vi "3D_to_2D_Sum_sub.vi"(1 "3D array":ext[][][](array[numeric])=array5x10x784[39200 elements]) -> (0 "2D_sum array":ext[][](array[numeric]))   [LabVIEW 2021]
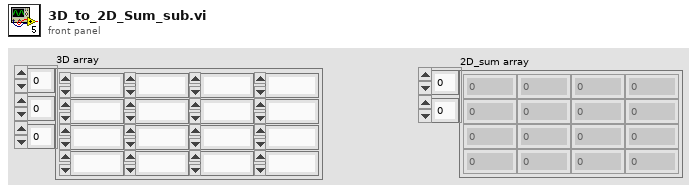
[diagram p1: front panel]
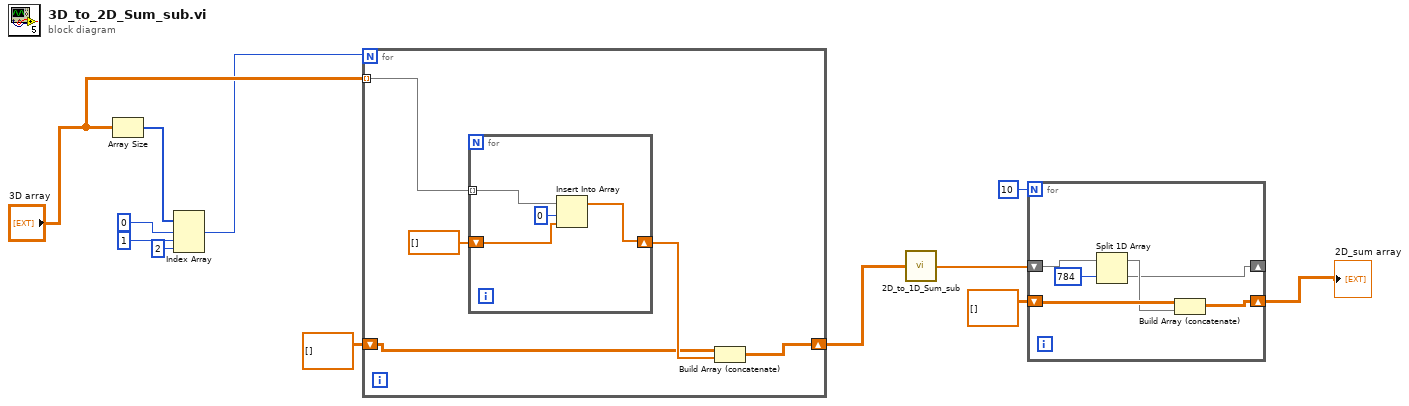
[diagram p0: block diagram]
diagram:
  n1 = Array Size(array="3D array") -> (size(s)=w12:i32[])
  n2 = Index Array(array=w12, index #1=0 ("인덱스"), index #2=1 ("인덱스"), index #3=2 ("인덱스")) -> (element #1=w7:i32)  [unwired: 2 out]
  n3 = for {
    N: w7 -> [_]
    tunnel: "3D array" -> [w16] mode=indexing
    shift-right: [w13] -> w5
    shift-left: ext[][] [] -> [w14]
    n4 = for {
      tunnel: w16 -> [w21] mode=indexing
      shift-right: [w20] -> w15
      shift-left: ext[] [] ("배열 2") -> [w19]
      n5 = Insert Into Array(array=w21, index=0 ("인덱스"), new element=w19) -> (w20:ext[])
    }
    n6 = Build Array (concatenate)(w14, w15) -> (w13:ext[][])
  }
  n7 = call "2D_to_1D_Sum_sub.vi"("2D array"=w5) -> ("1D array"=w2:ext[])
  n8 = for {
    N: 10 -> [_]
    shift-right: [w26] -> w1
    shift-left: dbl[][] [] -> [w25]
    shift-right: [w23] -> _
    shift-left: w2 -> [w22]
    n9 = Split 1D Array(array=w22, index=784) -> (first subarray=w24:ext[], second subarray=w23:ext[])
    n10 = Build Array (concatenate)(w25, w24) -> (w26:ext[][])
  }
  "2D_sum array" <- w1
